vi "VI Server_CycleEventBySignalingValue.vi"(7 "Label":string, 8 "error in":errorcluster, 11 "VI Server.RefsCluster":T1) -> (0 "error out":errorcluster, 3 "VI Server Cluster.DUP":T1)   [LabVIEW 2020, in "VI Server Toolkit LV2013.lvlib"]
doc: "Generates user event by specified control."
uses:
  VI Server Toolkit LV2013.lvlib
  VI Server_TypeDefs/VI Server_RefsCluster.ctl
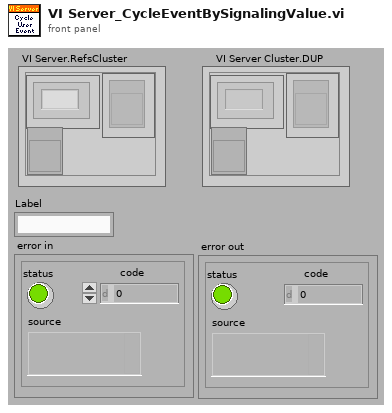
[diagram p1: front panel]
types:
  T1 = typedef "VI Server_RefsCluster.ctl" = cluster{"Labels":string[], "Refs":refnum<vi>[], "VI Ref":refnum<vi>}
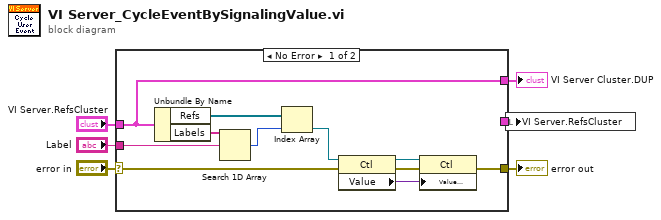
[diagram p0: block diagram]
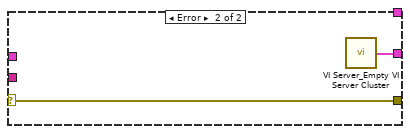
[diagram p2: hidden frame]
diagram:
  n1 = case shown="No Error" "error in" {
    selector: "error in" -> [w11 w19]
    tunnel: "Label" -> [w16 _]
    tunnel: "VI Server.RefsCluster" -> [w7 _]
    tunnel: [w13 w19] -> w6
    tunnel: [w7 _] -> w2
    tunnel: [_ w18] -> w1
    frame No Error {
      n2 = Unbundle By Name(w7) -> ("Refs"=w14:refnum<vi>[], "Labels"=w17:string[])
      n3 = Search 1D Array(1D array=w17, element=w16) -> (index of element=w15:i32)  [unwired: 1 out]
      n4 = Index Array(array=w14, index=w15) -> (element=w12:refnum<vi>)
      n5 = property class="Ctl"(reference=w12, error in=w11) -> (reference out=w9:refnum<vi>, error out=w10:errorcluster, "Value"=w8:variant)
      n6 = property class="Ctl"(reference=w9, error in=w10, "Value (Signaling)"=w8) -> (error out=w13:errorcluster)  [unwired: 1 out]
    }
    frame Error {
      n7 = call "VI Server_Empty VI Server Cluster.vi"() -> ("VI Server Cluster"=w18:T1)  [unwired: 7 in]
    }
  }
  "error out" <- w6
  "VI Server Cluster.DUP" <- w2
  n8 = local write "VI Server.RefsCluster"(w1) -> ()
